vi "Ping.vi"(8 "error in (no error)":errorcluster, 10 "Queue":refnum<queue>, 11 "CO2 Actor in":refnum<class "CO2 Actor.lvclass">) -> (0 "error out":errorcluster, 3 "CO2 Actor out":refnum<class "CO2 Actor.lvclass">)   [LabVIEW 2015, in "cRIO-Carbondioxide.lvlib" / "CO2-Actor.lvlib" / "CO2 Actor.lvclass"]
uses:
  CO2 Actor.lvclass
  <vilib>/ActorFramework/Actor/Actor.lvclass
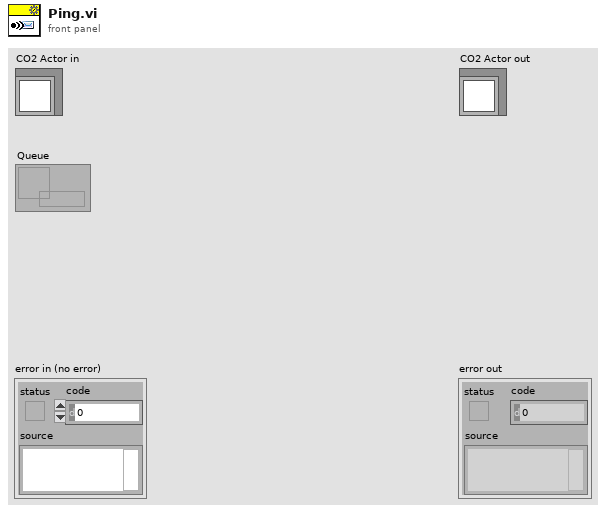
[diagram p1: front panel]
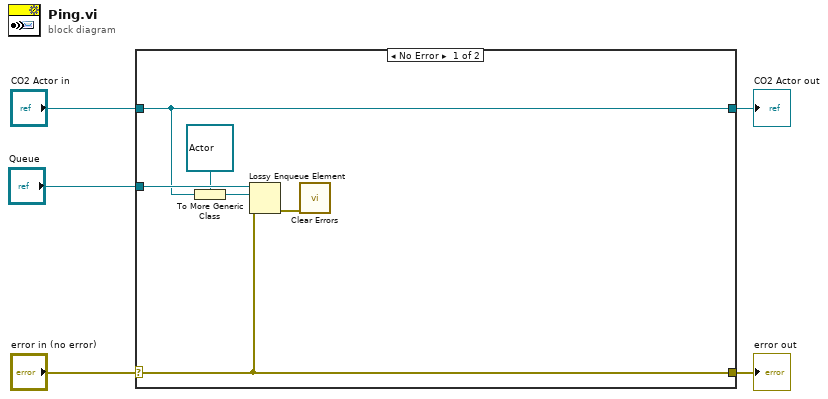
[diagram p0: block diagram]
diagram:
  n1 = case shown="No Error" "error in (no error)" {
    selector: "error in (no error)" -> [w6 w13]
    tunnel: [w6 w13] -> w4
    tunnel: [w10 w12] -> w2
    tunnel: "CO2 Actor in" -> [w10 w12]
    tunnel: "Queue" -> [w11 _]
    frame No Error {
      n2 = To More Generic Class(target class=refnum<class "Actor.lvclass"> refnum ("element"), reference=w10) -> (generic class reference=w8:refnum<class "Actor.lvclass">)
      n3 = Lossy Enqueue Element(queue=w11, element=w8, error in (no error)=w6) -> (error out=w7:errorcluster)  [unwired: 3 out]
      n4 = call <vilib>:"Clear Errors.vi"("error in (no error)"=w7) -> ()  [unwired: 5 in, 2 out]
    }
    frame Error {
    }
  }
  "error out" <- w4
  "CO2 Actor out" <- w2
